vi "RobotDLLToolEngage (SubVI).vi"(3 "Tool Insertion":bool, 4 "Tool Fast Retraction":bool, 5 "Target Tool Insertion Length":dbl, 6 "ArmID":i32, 7 "Target Tool Insertion Speed":dbl, 10 "Tool Withdraw":bool, 11 "Target Tool Withdraw Length":dbl, 12 "Target Tool Withdraw Speed":dbl) -> (0 "actInsertionLength":dbl)   [LabVIEW 2016]
uses:
  EyeRobotDLL.dll
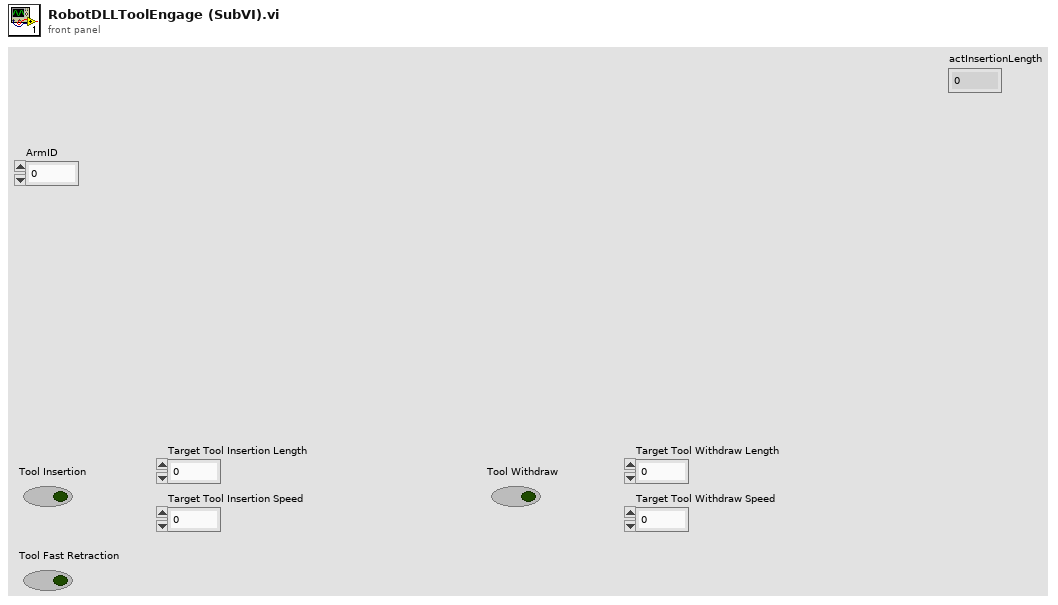
[diagram p1: front panel]
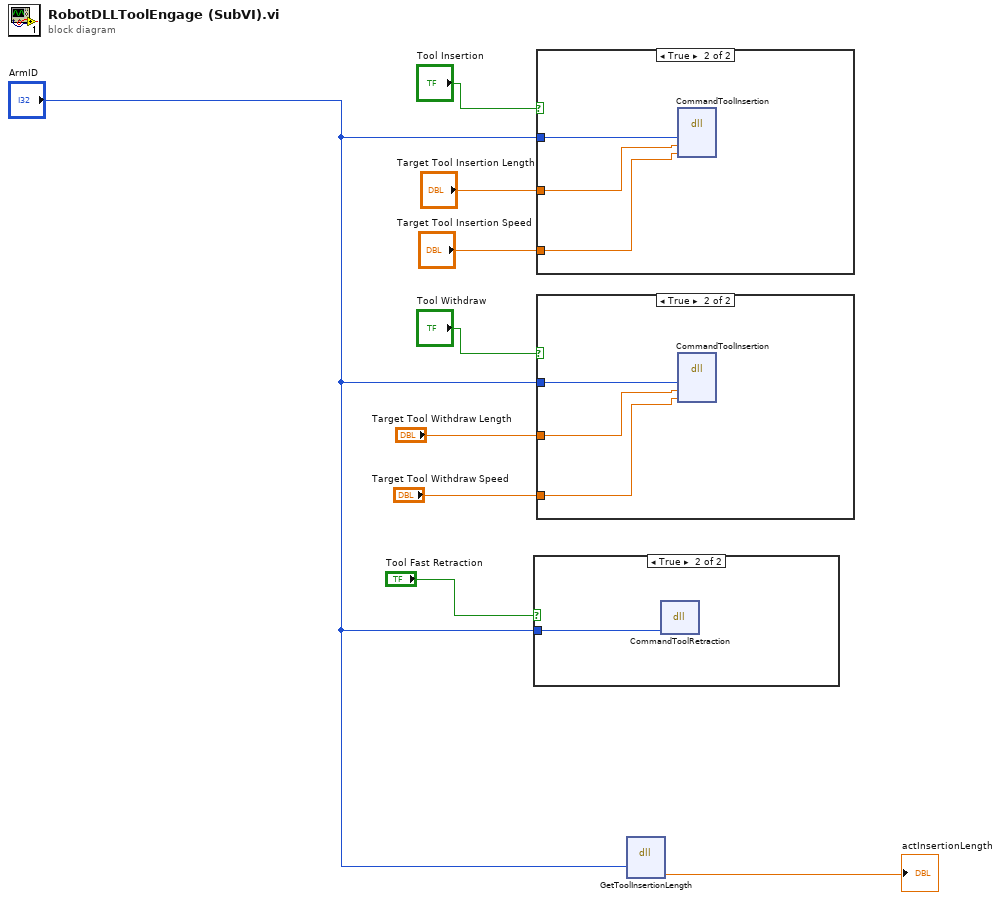
[diagram p0: block diagram]
diagram:
  n1 = case shown="True" "Tool Fast Retraction" {
    tunnel: "ArmID" -> [_ w10]
    frame False {
    }
    frame True {
      n2 = dll-call lib="D:/Kevin/IRISSoft LV2016 dev/Host Demo/Functions/EyeRobotDLL.dll" fn="CommandToolRetraction"("id"=w10) -> ()  [unwired: 5 in, 2 out]
    }
  }
  n3 = case shown="True" "Tool Insertion" {
    tunnel: "ArmID" -> [_ w13]
    tunnel: "Target Tool Insertion Length" -> [_ w12]
    tunnel: "Target Tool Insertion Speed" -> [_ w11]
    frame False {
    }
    frame True {
      n4 = dll-call lib="D:/Kevin/IRISSoft LV2016 dev/Host Demo/Functions/EyeRobotDLL.dll" fn="CommandToolInsertion"("id"=w13, "insertionLength"=w12, "speed"=w11) -> ()  [unwired: 7 in, 2 out]
    }
  }
  n5 = case shown="True" "Tool Withdraw" {
    tunnel: "ArmID" -> [_ w16]
    tunnel: "Target Tool Withdraw Length" -> [_ w15]
    tunnel: "Target Tool Withdraw Speed" -> [_ w14]
    frame False {
    }
    frame True {
      n6 = dll-call lib="D:/Kevin/IRISSoft LV2016 dev/Host Demo/Functions/EyeRobotDLL.dll" fn="CommandToolInsertion"("id"=w16, "insertionLength"=w15, "speed"=w14) -> ()  [unwired: 7 in, 2 out]
    }
  }
  n7 = dll-call lib="D:/Kevin/IRISSoft LV2016 dev/Host Demo/Functions/EyeRobotDLL.dll" fn="GetToolInsertionLength"("id"="ArmID") -> ("insertionLength"=→"actInsertionLength":dbl)  [unwired: 6 in, 2 out]
